vi "heat_laser_calibration.vi"(0 "heat_board_control.lvclass":refnum<class "heat_board_control.lvclass">, 1 "Cluster":T1, 2 "Lock-in parameters":T3={"frequency"=1000.0, "order"=3, "low cutoff freq: fl"=200.0} {"low cutoff freq: fl" format="%#_13g"; "frequency" format="%0.2p"}, 3 "error in (no error)":errorcluster, 4 "sampling info":cluster{"Fs":dbl, "#s":dbl}={"Fs"=5000.0, "#s"=1000.0} {"Fs" format="%.2p"}) -> (6 "percent done":dbl(knob) scale=0.0..100.0, 7 "heat_board_control out 2":refnum<class "heat_board_control.lvclass">, 8 "best setpoint":dbl, 9 "Waveform Chart":dbl(graph), 10 "error out":errorcluster)   [LabVIEW 2015]
uses:
  heat_board_control.lvclass
  <vilib>/Analysis/baseanly.llb/Mean (DBL).vi
  <vilib>/ULx/Write.llb/ULx Write (Analog 1D DBL 1Chan 1Samp).vi
  <vilib>/Analysis/NI_AALBase.lvlib
panel:
  in  "sweep parameters":T2={"start point"=1.0, "end point"=2.0, "increment"=0.01, "delay time (s)"=0.5}
  # "Locks into frequency to find modulation amplitude"
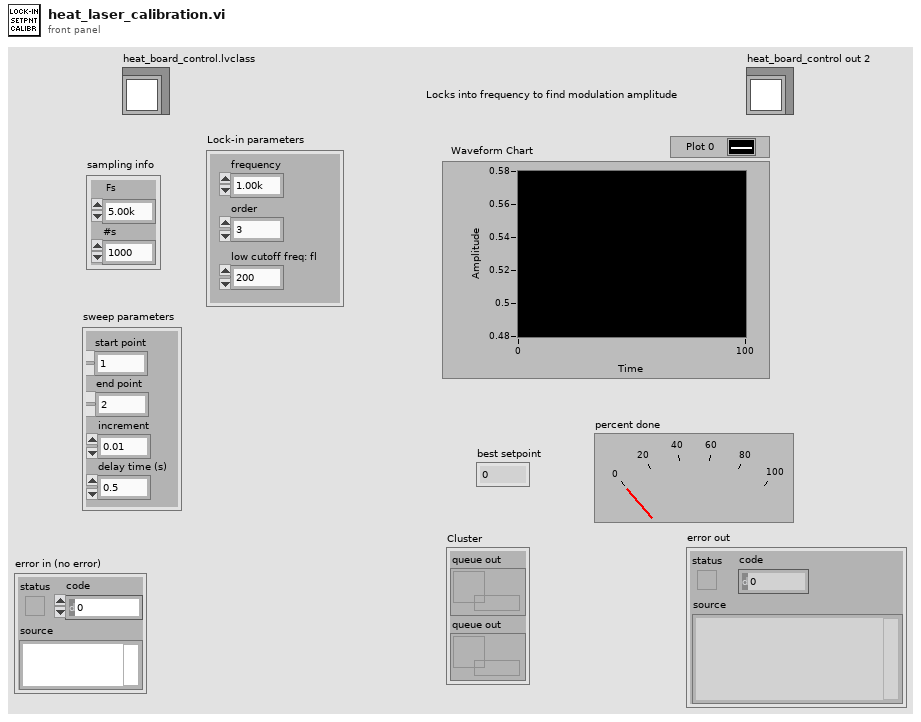
[diagram p1: front panel]
types:
  T1 = cluster{"queue out":refnum<queue>, "queue out":refnum<queue>}
  T2 = cluster{"start point":dbl, "end point":dbl, "increment":dbl, "delay time (s)":dbl}
  T3 = cluster{"frequency":dbl, "order":i32, "low cutoff freq: fl":dbl}
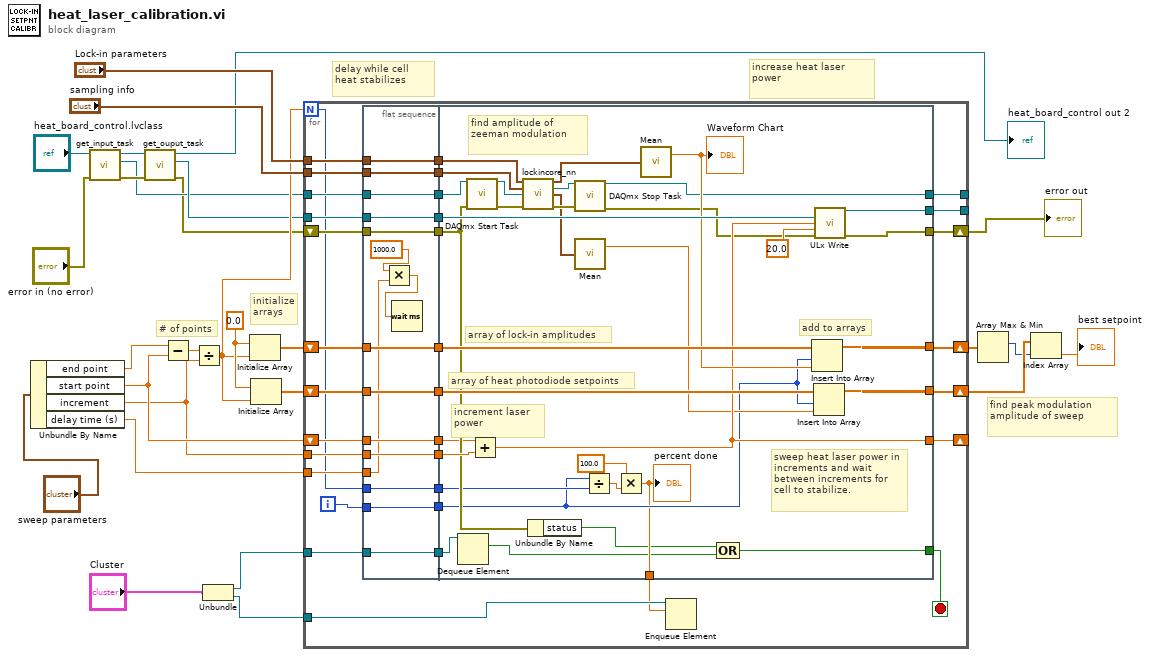
[diagram p0: block diagram]
diagram:
  w23 = 0.0 ("element")
  # "# of points"
  # "initialize\narrays"
  # "delay while cell heat stabilizes"
  # "increase heat laser power"
  # "find peak modulation amplitude of sweep"
  n1 = Unbundle By Name("sweep parameters") -> ("end point"=w15:dbl, "start point"=w14:dbl, "increment"=w13:dbl, "delay time (s)"=w12:dbl)
  n2 = call-dynamic "get_input_task.vi"("error in (no error)"="error in (no error)", "heat_board_control in"="heat_board_control.lvclass") -> ("error out"=w8:errorcluster, "input task out"=w5:refnum<k21>, "heat_board_control out"=w9:refnum<class "heat_board_control.lvclass">)  [unwired: 7 in]
  n3 = call-dynamic "get_ouput_task.vi"("error in (no error)"=w8, "heat_board_control in"=w9) -> ("error out"=w4:errorcluster, "output task out"=w10:refnum<k24>, "heat_board_control out"=→"heat_board_control out 2":refnum<class "heat_board_control.lvclass">)  [unwired: 7 in]
  n4 = Subtract(x=w15, y=w14) -> (x-y=w26:dbl)
  n5 = Divide(x=w26, y=w13) -> (x/y=w18:dbl)
  n6 = Unbundle("Cluster") -> ("queue out"=w2:refnum<queue>, "queue out"=w3:refnum<queue>)
  n7 = Initialize Array(w23, w18) -> (w25:dbl[])
  n8 = Initialize Array(w23, w18) -> (w22:dbl[])
  n9 = for {
    N: w18 -> [w34]
    tunnel: "sampling info" -> [w59]
    shift-right: [w48] -> w17
    shift-left: w4 -> [w62]
    tunnel: "Lock-in parameters" -> [w58]
    tunnel: w12 -> [w53]
    shift-right: [w52] -> w24
    shift-left: w25 -> [w51]
    shift-right: [w50] -> w21
    shift-left: w22 -> [w49]
    tunnel: w5 -> [w60]
    tunnel: [w61] -> _
    tunnel: w10 -> [w57]
    tunnel: [w56] -> _
    tunnel: w13 -> [w54]
    shift-right: [w47] -> _
    shift-left: w14 -> [w55]
    tunnel: w3 -> [w32]
    tunnel: w2 -> [w30]
    i -> [w37]
    stop <- w35 stop-if-true
    n10 = flat-sequence {
      tunnel: w49 -> [w69]
      tunnel: w51 -> [w70]
      tunnel: w53 -> [w65]
      tunnel: w54 -> [w71]
      tunnel: w55 -> [w72]
      tunnel: w57 -> [w73]
      tunnel: w58 -> [w74]
      tunnel: w59 -> [w75]
      tunnel: w60 -> [w76]
      tunnel: w62 -> [w77]
      tunnel: [w77] -> w46
      tunnel: [w76] -> w45
      tunnel: [w75] -> w44
      tunnel: [w74] -> w43
      tunnel: [w73] -> w42
      tunnel: [w72] -> w41
      tunnel: [w71] -> w40
      tunnel: [w70] -> w39
      tunnel: [w69] -> w38
      tunnel: w37 -> [w67]
      tunnel: [w67] -> w36
      tunnel: w34 -> [w64]
      tunnel: [w64] -> w33
      tunnel: w30 -> [w63]
      tunnel: [w63] -> w29
      tunnel: [w94] -> w61
      tunnel: [w106] -> w56
      tunnel: [w104] -> w52
      tunnel: [w101] -> w50
      tunnel: [w99] -> w48
      tunnel: [w98] -> w47
      tunnel: w46 -> [w90]
      tunnel: w45 -> [w91]
      tunnel: w44 -> [w111]
      tunnel: w43 -> [w109]
      tunnel: w42 -> [w107]
      tunnel: w41 -> [w87]
      tunnel: w40 -> [w105]
      tunnel: w39 -> [w103]
      tunnel: w38 -> [w100]
      tunnel: w36 -> [w85]
      tunnel: [w79] -> w35
      tunnel: w33 -> [w86]
      tunnel: [w82] -> w31
      tunnel: w29 -> [w78]
      frame #0 {
        n11 = Multiply(x=1000.0 ("y"), y=w65) -> (x*y=w68:dbl)
        n12 = Wait (ms)(milliseconds to wait=w68) -> ()  [unwired: 1 out]
      }
      frame #1 {
        # "increment laser power"
        # "add to arrays"
        # "array of heat photodiode setpoints"
        # "array of lock-in amplitudes"
        # "find amplitude of zeeman modulation"
        # "sweep heat laser power in increments and wait between increments for cell to stabilize."
        n13 = Dequeue Element(queue=w78) -> (element=w81:bool)  [unwired: 2 in, 3 out]
        n14 = call <vilib>:"DAQmx Start Task.vi"("task/channels in"=w91, "error in"=w90) -> ("task out"=w92:refnum<k21>, "error out"=w93:errorcluster)  [unwired: 12 in]
        n15 = Add(x=w87, y=w105) -> (x+y=w98:dbl)
        n16 = call "lockincore_nn.vi"("Lock-in parameters"=w109, "sampling info"=w111, "task/channels in"=w92, "error in (no error)"=w93) -> ("lock-in"=w110:waveform(dbl), "task out"=w95:refnum<k21>, "photodiode"=w89:waveform(dbl), "error out"=w97:errorcluster)  [unwired: 8 in]
        n17 = Unbundle By Name(w90) -> ("status"=w80:bool)
        n18 = call <vilib>:"DAQmx Stop Task.vi"("task/channels in"=w95, "error in"=w97) -> ("task out"=w94:refnum<k21>, "error out"=w96:errorcluster)  [unwired: 12 in]
        n19 = call-poly <vilib>:"Mean.vi"("X"=w89) -> ("mean"=w88:dbl)  [unwired: 1 out]
        n20 = Divide(x=w85, y=w86) -> (x/y=w84:dbl)
        n21 = Multiply(x=100.0, y=w84) -> (x*y=w82:dbl)
        "percent done" <- w82
        n22 = call-poly <vilib>:"Mean.vi"("X"=w110) -> ("mean"=w102:dbl)  [unwired: 1 out]
        "Waveform Chart" <- w102
        n23 = Compound Arithmetic op=OR(w80, w81) -> (w79:bool)
        n24 = Insert Into Array(array=w103, index=w85, new element=w102) -> (w104:dbl[])
        n25 = Insert Into Array(array=w100, index=w85, new element=w88) -> (w101:dbl[])
        n26 = call-poly <vilib>:"ULx Write.vi"("task in"=w107, "data"=w98, "timeout"=20.0, "error in"=w96) -> ("task out"=w106:refnum<k24>, "error out"=w99:errorcluster)  [unwired: 9 in, 1 out]
      }
    }
    n27 = Enqueue Element(queue=w32, element=w31) -> ()  [unwired: 2 in, 3 out]
  }
  "error out" <- w17
  n28 = Array Max & Min(array=w24) -> (max index (indices)=w20:i32)  [unwired: 3 out]
  n29 = Index Array(array=w21, index=w20) -> (element=→"best setpoint":dbl)
